vi "Hardware-EPTxData.vi"(11 "DCM Ref":refnum<class "DCM - RT.lvclass">) -> (3 "EPTxData":T1)   [LabVIEW 2016, in "DSI-RT.lvlib"]
uses:
  DSI-RT.lvlib
  <vilib>/Powertrain Controls/Device Drivers/Engine Position Tracking/EPTx/RevA/RT/Controls/EPTxData.ctl
  <vilib>/Powertrain Controls/Device Drivers/DCM/Rev0/RT/DCM - RT.lvclass
  <vilib>/Powertrain Controls/Device Drivers/DCM/Rev0/RT/DCM - RT.lvclass/DCM - RT.ctl
  <vilib>/Powertrain Controls/Device Drivers/DCM/Rev0/RT/Read FPGA Reference.vi
  <vilib>/Utility/error.llb/Error Cluster From Error Code.vi
  <vilib>/rvi/errors/niLvFpgaAdjustHostInterfaceError.vi
  <vilib>/rvi/interface/nirviReadWriteControl/nirviReadWriteControl.xnode
  <vilib>/Powertrain Controls/Device Drivers/Engine Position Tracking/EPTx/RevA/RT/EPTx - RevA - RT.lvlib
  NiFpgaLv.dll
  <vilib>/rvi/interface/Simulation/niFpgaSimulationCallBeginRW.vi
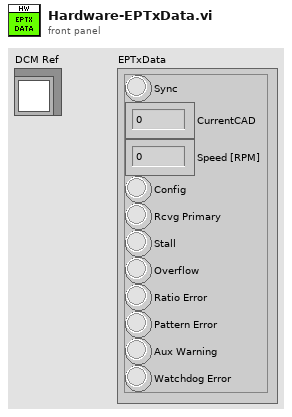
[diagram p1: front panel]
types:
  T1 = typedef "EPTx - RevA - RT.lvlib/EPTxData.ctl" = cluster{"Sync":bool, "CurrentCAD":sgl, "Speed [RPM]":sgl, "Config":bool, "Rcvg Primary":bool, "Stall":bool, "Overflow":bool, "Ratio Error":bool, "Pattern Error":bool, "Aux Warning":bool, "Watchdog Error":bool}
  T2 = cluster{"Sync":bool, "CurrentCAD":fxp<+,18,11>, "MaxCAD":fxp<+,11,11>, "HistoryCAD":fxp<+,11,11>, "CADRate":fxp<+,22,8>, "AvgSpeed":fxp<+,17,15>, "Config":bool, "Rcvg Primary":bool, "Stall":bool, "Overflow":bool, "Ratio Error":bool, "Pattern Error":bool, "Aux Warning":bool, "Watchdog Error":bool}
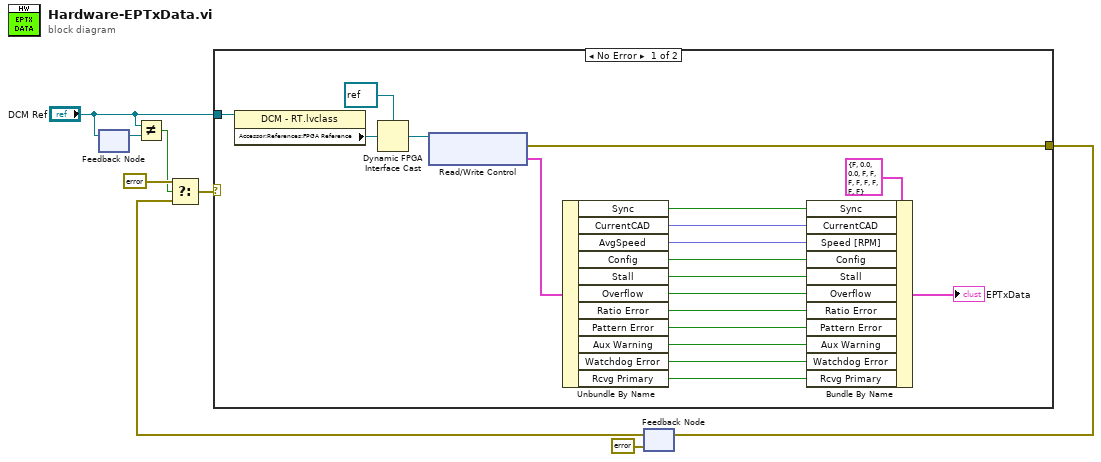
[diagram p0: block diagram]
diagram:
  n1 = feedback #1() -> (w3:refnum<class "DCM - RT.lvclass">)  [unwired: 1 in]
  n2 = feedback-in #1("DCM Ref") -> ()
  n3 = Not Equal?(x="DCM Ref", y=w3) -> (x != y?=w1:bool)
  n4 = feedback #2(errorcluster {"status"=FALSE, "code"=0, "source"=""} ("error out")) -> (w5:errorcluster)
  n5 = Select(t=errorcluster {"status"=FALSE, "code"=0, "source"=""}, s=w1, f=w5) -> (s? t:f=w7:errorcluster)
  n6 = case shown="No Error" w7 {
    selector: w7 -> [_ w28]
    tunnel: "DCM Ref" -> [w13 _]
    tunnel: [w9 w28] -> w6
    frame No Error {
      n7 = property class="DCM - RT.lvclass"(reference=w13) -> ("Accessor:References:FPGA Reference"=w12:refnum<k20>)  [unwired: 1 in, 2 out]
      n8 = Dynamic FPGA Interface Cast(Session In=refnum<k20> refnum ("FPGA VI Reference"), Type=w12) -> (Session Out=w10:refnum<k20>)
      n9 = xnode ("Read/Write Control")("FPGA VI Reference In"=w10) -> ("error out"=w9:errorcluster, "EPTxSupervisor"=w14:T2)  [unwired: 1 in, 1 out]
      n10 = Unbundle By Name(w14) -> ("Sync"=w23:bool, "CurrentCAD"=w24:fxp<+,18,11>, "AvgSpeed"=w27:fxp<+,17,15>, "Config"=w17:bool, "Stall"=w18:bool, "Overflow"=w19:bool, "Ratio Error"=w20:bool, "Pattern Error"=w21:bool, "Aux Warning"=w22:bool, "Watchdog Error"=w25:bool, "Rcvg Primary"=w26:bool)
      n11 = Bundle By Name(cluster=T1 {"Sync"=FALSE, "CurrentCAD"=0.0, "Speed [RPM]"=0.0, "Config"=FALSE, "Rcvg Primary"=FALSE, "Stall"=FALSE, "Overflow"=FALSE, "Ratio Error"=FALSE, "Pattern Error"=FALSE, "Aux Warning"=FALSE, "Watchdog Error"=FALSE} ("EPTx Data"), "Sync"=w23, "CurrentCAD"=w24, "Speed [RPM]"=w27, "Config"=w17, "Stall"=w18, "Overflow"=w19, "Ratio Error"=w20, "Pattern Error"=w21, "Aux Warning"=w22, "Watchdog Error"=w25, "Rcvg Primary"=w26) -> (→"EPTxData":T1)
    }
    frame Error {
    }
  }
  n12 = feedback-in #2(w6) -> ()
